vi "AW.vi"(8 "Orifice_Plate_Diameter":dbl=13.0 format="%#_13g", 9 "Ambient_temperature":dbl=23.365 format="%#_13g", 10 "Box_Pressure":dbl=22.27 format="%#_13g", 11 "Ambient_Pressure":dbl=101.599 format="%#_13g") -> (1 "AP":dbl, 2 "Q":dbl)   [LabVIEW 2017]
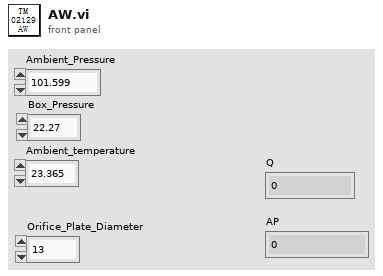
[diagram p1: front panel]
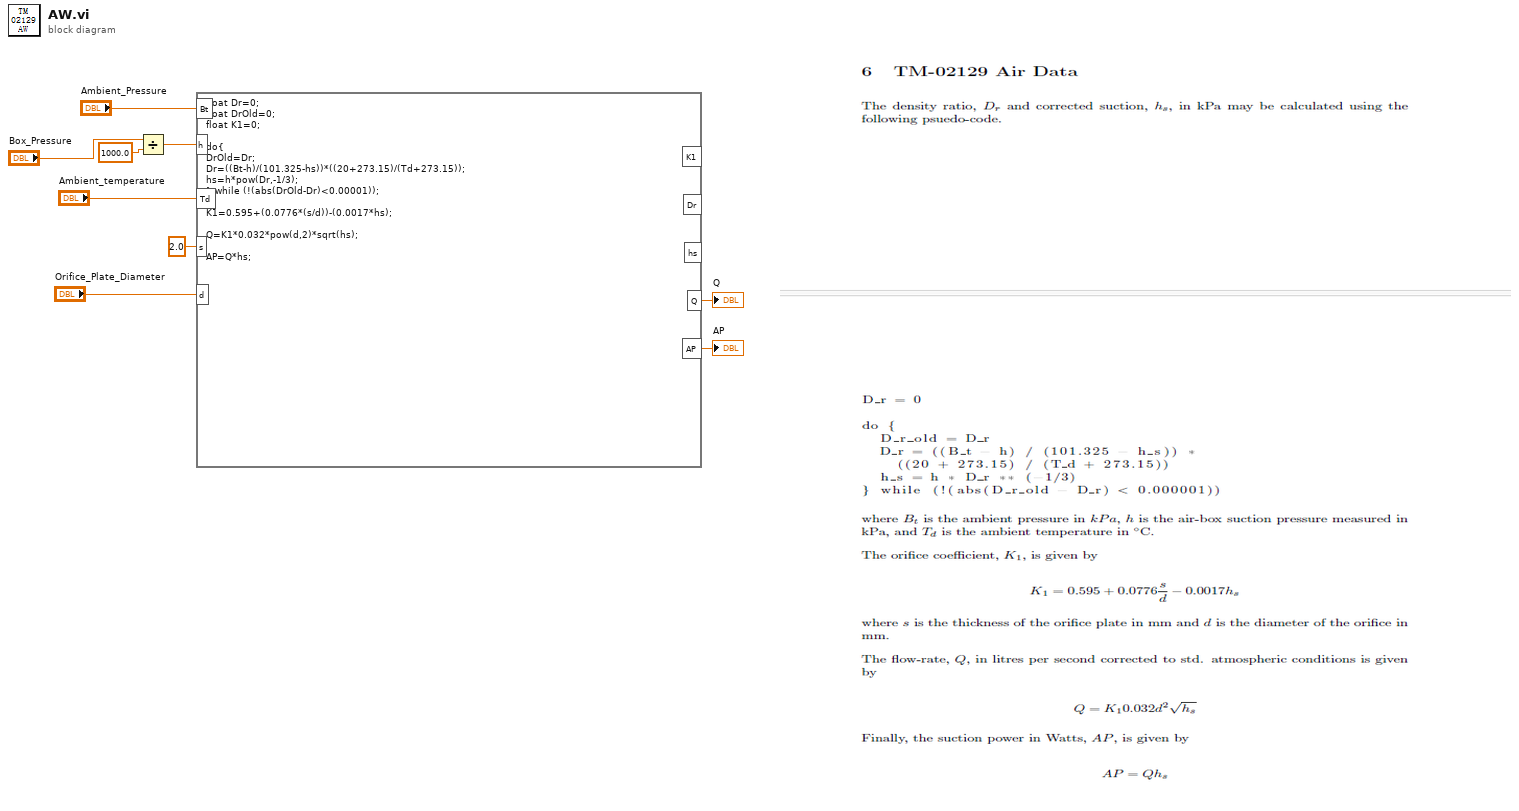
[diagram p0: block diagram]
diagram:
  n1 = Divide(x="Box_Pressure", y=1000.0) -> (x/y=w4:dbl)
  n2 = formula code="float Dr=0;\nfloat DrOld=0;\nfloat K1=0;\n\ndo{\nDrOld=Dr;\nDr=((Bt-h)/(101.325-hs))*((20+273.15)/(Td+273.15));\nhs=h*pow(Dr,-1/3);\n} while (!(abs(DrOld-Dr)<0.00001));\n\nK1=0.595+(0.0776*(s/d))-(0.0017*hs);\n\nQ=K1*0.032*pow(d,2)*sqrt(hs);\n\nAP=Q*hs;"("s"=2.0 ("输入变量"), "Td"="Ambient_temperature", "Bt"="Ambient_Pressure", "h"=w4, "d"="Orifice_Plate_Diameter") -> ("Q"=→"Q":dbl, "AP"=→"AP":dbl)  [unwired: 3 out]
